vi "HostMain.vi"() -> ()   [LabVIEW 2012]
uses:
  Support VIs/operationModes.ctl
  <vilib>/MakerHub/KinectOne/Private/Type Defs/BodyData.ctl
  <vilib>/MakerHub/KinectOne/Private/Type Defs/ClippedEdges.ctl
  <vilib>/MakerHub/KinectOne/Private/Type Defs/HandLeftConfidence.ctl
  <vilib>/MakerHub/KinectOne/Private/Type Defs/HandLeftState.ctl
  <vilib>/MakerHub/KinectOne/Private/Type Defs/HandRightConfidence.ctl
  <vilib>/MakerHub/KinectOne/Private/Type Defs/HandRightState.ctl
  Microsoft.Kinect
  <vilib>/MakerHub/KinectOne/Private/Type Defs/LeanTrackingState.ctl
  Messages.ctl
  Support VIs/messageTypes.ctl
  GainsTDef.ctl
  Support VIs/speeds.ctl
  PolarCoordTdef.ctl
  Support VIs/setpointCluster.ctl
  StopTDef.ctl
  <vilib>/MakerHub/PS4-Controller/Public/Open First Controller.vi
  <vilib>/MakerHub/KinectOne/Private/Initialize Image [Color].vi
  <vilib>/MakerHub/KinectOne/Private/kinectRead [ColorFrame].vi
  <vilib>/MakerHub/KinectOne/Private/kinectRead [BodyFrame].vi
  <vilib>/MakerHub/KinectOne/KinectOne.lvlib
  <vilib>/MakerHub/PS4-Controller/LMH-PS4.lvlib
panel:
  in  "colour mode (T = dist, F = sphere)":bool
  out "Detected Colour":u32(colorbox)
  out "Tracked?":bool
  in  "Forward Speed Limit [rad/s] (10 r/s)":dbl(knob)=2.995028509599303 scale=0.0..10.0
  out "Parameter Closed":bool
  out "Kinect Closed":bool
  out "Ctrl Event Loop Off":bool
  out "Controller Off":bool
  out "Hand Ctrl Closed":bool
  out "Message Sender Closed":bool
  in  "ControllerStop":bool
  out "Controller?":bool
  out "Toggle":bool
  in  "Skynet\nButton":bool
  out "TX":bool
  in  "bodyData":T1[](array[typedef])
  in  "Modulus SP":dbl=1.7999999523162842
  in  "Reference\nColour":u32(colorbox)
  in  "Argument SP":dbl
  out "index":i32
  in  "Operation Mode":T8 items=["TeleOp", "Desperate", "ColourMatch"]
  out "Image":T9(plugin-control)
  in  "Kd-Argument":dbl
  in  "Kc-Argument":dbl=0.30000001192092896
  in  "Kd-Modulus":dbl
  in  "Kc-Modulus":dbl=0.5
  out "Mod":dbl
  out "Arg":dbl
  in  "Program Stop":bool
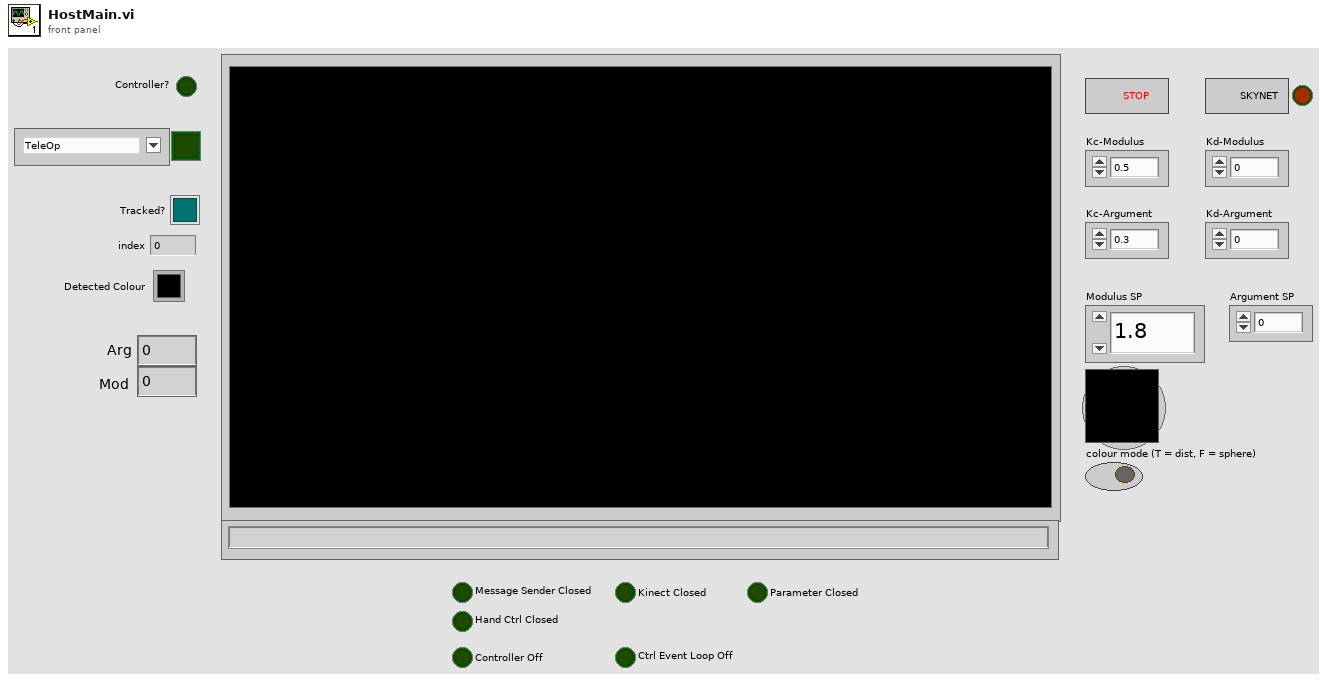
[diagram p1: front panel]
types:
  T1 = typedef "KinectOne.lvlib/BodyData.ctl" = cluster{"ClippedEdges":T2, "HandLeftConfidence":T3, "HandLeftState":T4, "HandRightConfidence":T5, "HandRightState":T6, "IsRestricted":bool, "IsTracked":bool, "JointOrientations":refnum<k24>, "Joints":refnum<k24>, "Lean":refnum<k24>, "LeanTrackingState":T7, "TrackingId":u64}
  T2 = typedef "KinectOne.lvlib/ClippedEdges.ctl" = enum16{"None", "Right", "Left", "Top", "Bottom"}
  T3 = typedef "KinectOne.lvlib/HandLeftConfidence.ctl" = enum16{"Low", "High"}
  T4 = typedef "KinectOne.lvlib/HandLeftState.ctl" = enum16{"Unknown", "NotTracked", "Open", "Closed", "Lasso"}
  T5 = typedef "KinectOne.lvlib/HandRightConfidence.ctl" = enum16{"Low", "High"}
  T6 = typedef "KinectOne.lvlib/HandRightState.ctl" = enum16{"Unknown", "NotTracked", "Open", "Closed", "Lasso"}
  T7 = typedef "KinectOne.lvlib/LeanTrackingState.ctl" = enum16{"NotTracked", "Inferred", "Tracked"}
  T8 = typedef "operationModes.ctl" = u16
  T9 = typedef "IMAQ Image.ctl" = refnum<image>
  T10 = typedef "GainsTDef.ctl" = cluster{"Kp-Modulus":dbl, "Kd-Modulus":dbl, "Kp-Argument":dbl, "Kd-Argument":dbl}
  T11 = typedef "Messages.ctl" = cluster{"message data":variant, "message type":T12}
  T12 = typedef "messageTypes.ctl" = enum16{"Speeds", "Stop", "PolarCoordinates", "Gains", "Setpoints"}
  T13 = typedef "KinectOne.lvlib/KinectSensor References.ctl" = cluster{"KinectSensor":refnum<k24>, "MultiSourceFrameReader":refnum<k24>, "BodyFrameDataInterface":refnum<k24>}
  T14 = typedef "LMH-PS4.lvlib/PS4 Controller Ref.ctl" = cluster{"Controller Ref":refnum<k1>, "PS4 Events Ref":refnum<event-registration>, "Worker Ref":refnum<vi>}
  T15 = typedef "speeds.ctl" = cluster{"left motor [rad/s]":dbl, "right motor [rad/s]":dbl}
  T16 = typedef "PolarCoordTdef.ctl" = cluster{"Argument":dbl, "Modulus":dbl, "trackedState":bool}
  T17 = typedef "KinectOne.lvlib/Joint Position.ctl" = cluster{"Camera Space":cluster{"X":dbl, "Y":dbl, "Z":dbl}, "Color Space":cluster{"X":dbl, "Y":dbl}, "Depth Space":cluster{"X":dbl, "Y":dbl}, "Tracking State":enum16{"NotTracked", "Inferred", "Tracked"}}
  T18 = typedef "setpointCluster.ctl" = cluster{"Modulus Setpoint":dbl, "Argument Setpoint":dbl}
  T19 = typedef "StopTDef.ctl" = cluster{"stop":bool}
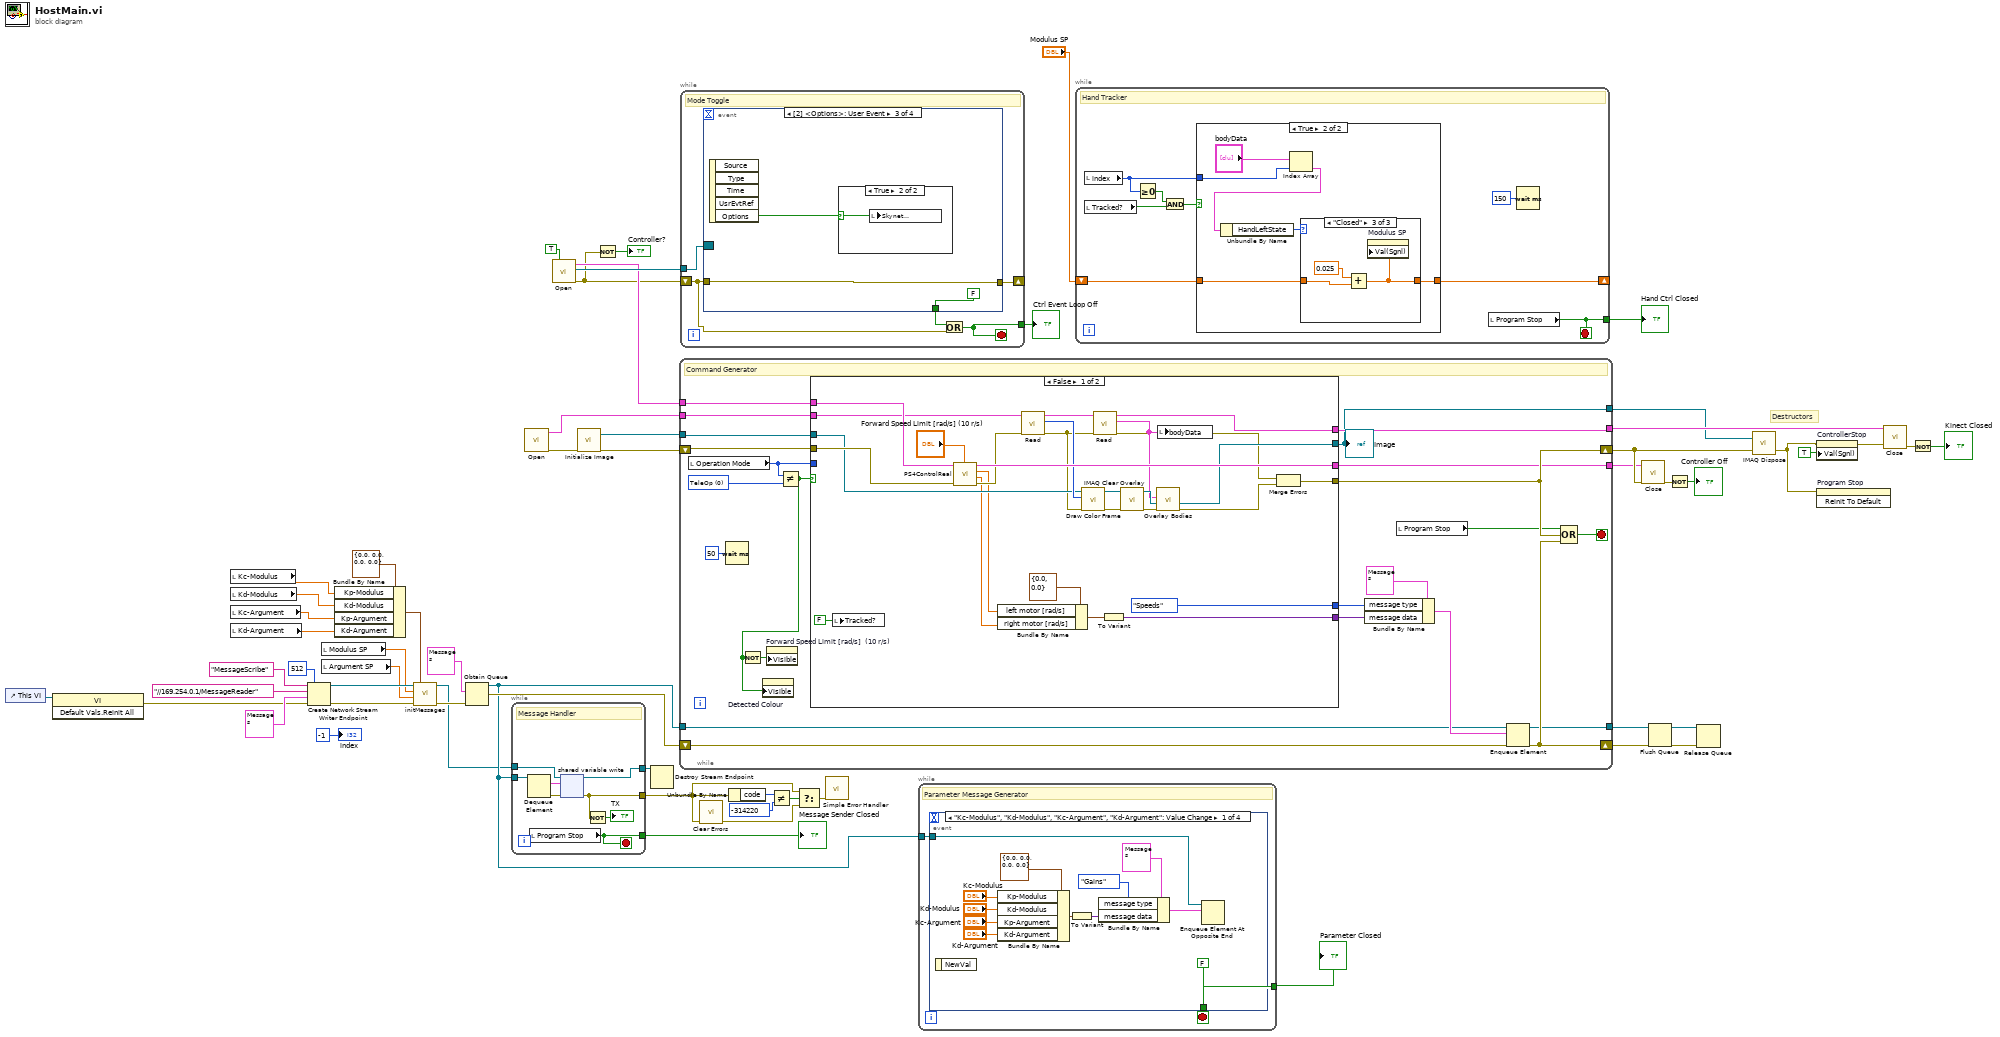
[diagram p0: block diagram]
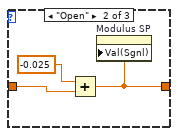
[diagram p4: hidden frame]
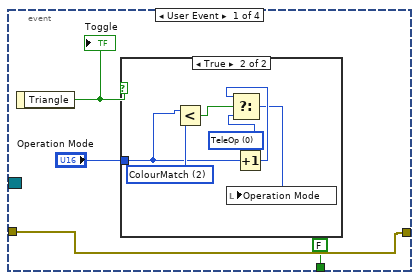
[diagram p5: hidden frame]
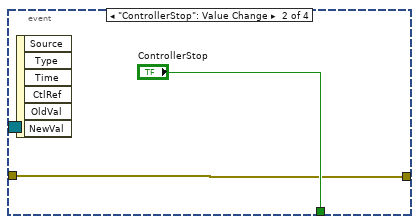
[diagram p7: hidden frame]
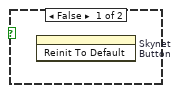
[diagram p8: hidden frame]
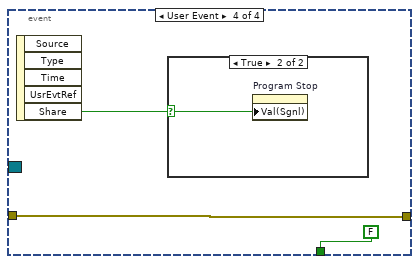
[diagram p9: hidden frame]
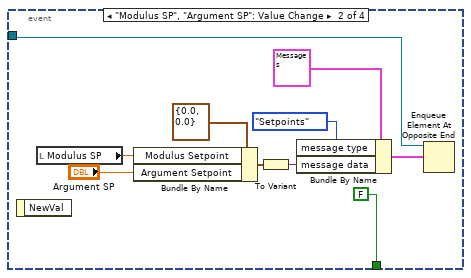
[diagram p11: hidden frame]
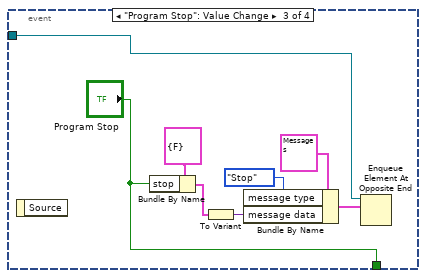
[diagram p12: hidden frame]
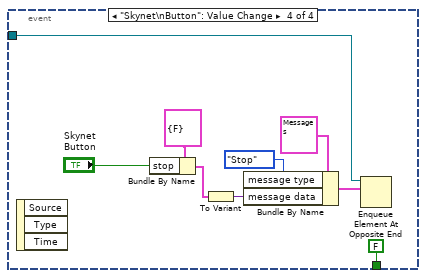
[diagram p13: hidden frame]
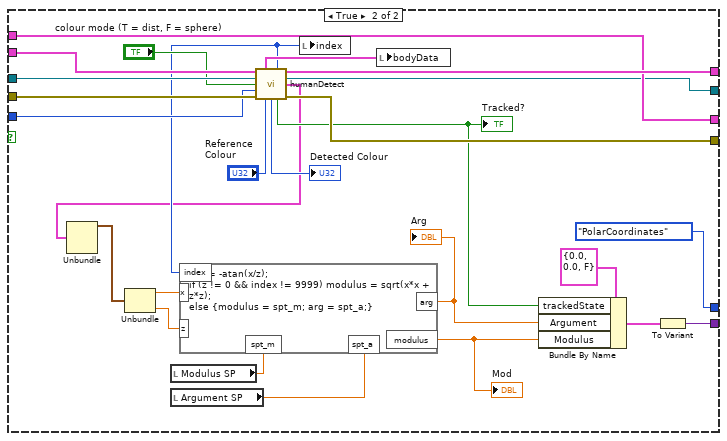
[diagram p14: hidden frame]
diagram:
  # "Destructors"
  n1 = control-ref of="This VI"() -> (w7:refnum<vi>)
  n2 = invoke class="VI" method="Default Vals.Reinit All"(reference=w7) -> (error out=w2:errorcluster)  [unwired: 2 in, 2 out]
  n3 = local read "Kc-Modulus"() -> (w30:dbl)
  n4 = local read "Kd-Modulus"() -> (w29:dbl)
  n5 = local read "Kc-Argument"() -> (w28:dbl)
  n6 = local read "Kd-Argument"() -> (w27:dbl)
  n7 = Create Network Stream Writer Endpoint(7:512 ("writer buffer size"), 8:w2, 9:T11 {"message data"=variant, "message type"=enum."Setpoints"} ("message"), 10:"//169.254.0.1/MessageReader" ("reader url"), 11:"MessageScribe" ("writer name")) -> (0:w3:errorcluster, 3:w25:refnum<k21>)  [unwired: 2 in]
  n8 = local read "Modulus SP"() -> (w24:dbl)
  n9 = local read "Argument SP"() -> (w23:dbl)
  n10 = Bundle By Name(cluster=T10 {"Kp-Modulus"=0.0, "Kd-Modulus"=0.0, "Kp-Argument"=0.0, "Kd-Argument"=0.0}, "Kp-Modulus"=w30, "Kd-Modulus"=w29, "Kp-Argument"=w28, "Kd-Argument"=w27) -> (w26:T10)
  n11 = call "initMessages.vi"("GainsCluster"=w26, "error in (no error)"=w3, "Argument Setpoint"=w23, "Modulus Setpoint"=w24, "writer name in"=w25) -> ("error out"=w22:errorcluster, "Refnum out"=w21:refnum<k21>)  [unwired: 5 in]
  n12 = Obtain Queue(element data type=T11 {"message data"=variant, "message type"=enum."Stop"} ("message"), error in (no error)=w22) -> (queue out=w48:refnum<queue>, error out=w54:errorcluster)  [unwired: 3 in, 1 out]
  n13 = while {
    tunnel: w48 -> [w66]
    tunnel: [w64] -> w33
    tunnel: [w63] -> w32
    tunnel: w21 -> [w61]
    tunnel: [w60] -> w9
    stop <- w60 stop-if-true
    # "Message Handler"
    n14 = Dequeue Element(queue=w66) -> (element=w65:T11, error out=w59:errorcluster)  [unwired: 2 in, 2 out]
    n15 = local read "Program Stop"() -> (w60:bool)
    n16 = shared-variable-write(w61, w59, w65) -> (w64:refnum<k21>, w63:errorcluster)  [unwired: 1 in, 1 out]
    n17 = Not(x=w63) -> (.not. x?=→"TX":bool)
  }
  "Message Sender Closed" <- w9
  n18 = call <vilib>:"Open.vi"() -> ("Error Out"=w58:errorcluster, "KinectSensor References out"=w51:T13)  [unwired: 10 in]
  n19 = call-poly <vilib>:"Open.vi"("Enable Events (T)"=TRUE) -> ("Error Out"=w20:errorcluster, "Event Registration Refnum"=w52:refnum<event-registration>, "PS4 Controller Ref"=w50:T14)  [unwired: 8 in]
  n20 = call-poly <vilib>:"Initialize Image.vi"("Error In"=w58) -> ("Error Out"=w57:errorcluster, "Color Image"=w56:T9)  [unwired: 9 in]
  n21 = Not(x=w20) -> (.not. x?=→"Controller?":bool)
  n22 = Destroy Stream Endpoint(11:w33) -> ()  [unwired: 1 in, 1 out]
  n23 = while {
    tunnel: w51 -> [w84]
    tunnel: w56 -> [w83]
    shift-right: [w82] -> w15
    shift-left: w57 -> [w81]
    tunnel: [w80] -> w55
    tunnel: w48 -> [w85]
    tunnel: [w72] -> w45
    tunnel: w50 -> [w79]
    tunnel: [w78] -> w14
    shift-right: [w86] -> w44
    shift-left: w54 -> [w87]
    tunnel: [w67] -> w1
    stop <- w89 stop-if-true
    w74 = T8 0 items=["TeleOp", "Desperate", "ColourMatch"] ("y")
    # "Command Generator"
    n24 = local read "Operation Mode"() -> (w75:T8)
    n25 = Wait (ms)(milliseconds to wait=u32 50) -> ()  [unwired: 1 out]
    n26 = Not Equal?(x=w75, y=w74) -> (x != y?=w70:bool)
    n27 = Not(x=w70) -> (.not. x?=w69:bool)
    n28 = property on="Detected Colour" class="ColBox"("Visible"=w70) -> ()  [unwired: 2 in, 2 out]
    n29 = property on="Forward Speed Limit [rad/s]  (10 r/s)" class="Knob (strict)"("Visible"=w69) -> ()  [unwired: 2 in, 2 out]
    n30 = case shown="False" w70 {
      tunnel: w84 -> [w113 w140]
      tunnel: w83 -> [w111 w139]
      tunnel: [w91 w138] -> w82
      tunnel: w81 -> [w115 w137]
      tunnel: [w98 w136] -> w80
      tunnel: w79 -> [w116 w129]
      tunnel: [w114 w129] -> w78
      tunnel: w75 -> [_ w133]
      tunnel: [messageTypes."Speeds" ("message type") messageTypes."PolarCoordinates" ("message type")] -> w77
      tunnel: [w105 w131] -> w76
      tunnel: [w97 w117] -> w67
      frame False {
        n31 = local write "Tracked?"(FALSE) -> ()
        n32 = call "PS4ControlReal.vi"("Forward Speed Limit [rad/s] (10.7 r/s)"="Forward Speed Limit [rad/s] (10 r/s)", "Error In"=w115, "PS4 Controller Ref In"=w116) -> ("Error Out"=w110:errorcluster, "right motor out"=w108:dbl, "left motor out"=w109:dbl, "PS4 Controller Ref Out"=w114:T14)  [unwired: 5 in]
        n33 = Bundle By Name(cluster=T15 {"left motor [rad/s]"=0.0, "right motor [rad/s]"=0.0}, "left motor [rad/s]"=w109, "right motor [rad/s]"=w108) -> (w106:T15)
        n34 = call-poly <vilib>:"Read.vi"("Error In"=w110, "KinectSensor References in"=w113) -> ("Error Out"=w95:errorcluster, "frameData"=w112:u32[], "KinectSensor References out"=w99:T13)  [unwired: 7 in]
        n35 = call <vilib>:"Draw Color Frame.vi"("Error In"=w95, "U32 Array"=w112, "Image"=w111) -> ("Error Out"=w94:errorcluster, "Image Out"=w101:T9)  [unwired: 7 in]
        n36 = call-poly <vilib>:"Read.vi"("error in (no error)"=w95, "KinectSensor References in"=w99) -> ("error out"=w92:errorcluster, "Body Data"=w96:T1[], "KinectSensor References out"=w98:T13)  [unwired: 7 in]
        n37 = To Variant(anything=w106) -> (Variant=w105:variant)
        n38 = call "IMAQ Clear Overlay"("error in (no error)"=w94, "Image"=w101) -> ("error out"=w93:errorcluster, "Image Out"=w100:T9)  [unwired: 8 in]
        n39 = call <vilib>:"Overlay Bodies.vi"("Error In"=w93, "Image"=w100, "Body Data"=w96) -> ("Error Out"=w90:errorcluster, "Image Out"=w97:T9)  [unwired: 7 in]
        n40 = local write "bodyData"(w96) -> ()
        n41 = Merge Errors(w92, w90) -> (w91:errorcluster)
      }
      frame True {
        n42 = local read "Modulus SP"() -> (w123:dbl)
        n43 = local read "Argument SP"() -> (w135:dbl)
        n44 = call "humanDetect.vi"("KinectSensor References In"=w140, "Image Container"=w139, "Tolerance Mode"="colour mode (T = dist, F = sphere)", "Operation Mode"=w133, "Error In"=w137, "Reference Colour"="Reference\nColour") -> ("Body Data Out"=w128:T1[], "Index Out"=w124:i32, "KinectSensor References Out"=w136:T13, "Image Out"=w117:T9, "Joint Position Out"=w118:T17, "Averaged Colour"=→"Detected Colour":u32, "isTracked"=w127:bool, "Error Out"=w138:errorcluster)  [unwired: 2 in]
        "Tracked?" <- w127
        n45 = Unbundle(w118) -> ("Camera Space"=w142:cluster{"X":dbl, "Y":dbl, "Z":dbl})  [unwired: 3 out]
        n46 = Unbundle(w142) -> ("X"=w120:dbl, "Z"=w119:dbl)  [unwired: 1 out]
        n47 = formula code="arg = -atan(x/z);\nif (z != 0 && index != 9999) modulus = sqrt(x*x + z*z);\nelse {modulus = spt_m; arg = spt_a;}"("x"=w120, "z"=w119, "spt_m"=w123, "spt_a"=w135, "index"=w124) -> ("arg"=w122:dbl, "modulus"=w121:dbl)
        "Arg" <- w122
        "Mod" <- w121
        n48 = local write "index"(w124) -> ()
        n49 = local write "bodyData"(w128) -> ()
        n50 = Bundle By Name(cluster=T16 {"Argument"=0.0, "Modulus"=0.0, "trackedState"=FALSE}, "trackedState"=w127, "Argument"=w122, "Modulus"=w121) -> (w132:T16)
        n51 = To Variant(anything=w132) -> (Variant=w131:variant)
      }
    }
    "Image" <- w67
    n52 = Bundle By Name(cluster=T11 {"message data"=variant, "message type"=enum."Stop"} ("message"), "message type"=w77, "message data"=w76) -> (w88:T11)
    n53 = local read "Program Stop"() -> (w68:bool)
    n54 = Enqueue Element(queue=w85, element=w88, error in (no error)=w87) -> (queue out=w72:refnum<queue>, error out=w86:errorcluster)  [unwired: 1 in, 1 out]
    n55 = Compound Arithmetic op=OR(w68, w82, w86) -> (w89:bool)
  }
  n56 = while {
    tunnel: w52 -> [w147]
    tunnel: [w143] -> w10
    shift-right: [w146] -> _
    shift-left: w20 -> [w144]
    stop <- w143 stop-if-true
    # "Mode Toggle"
    n57 = event shown="[2] <Options>: User Event" {
      selector: w147 -> [_ _ _ _]
      dyn-events: _ -> [_ _ _ _]
      timeout: _ -> [_ _ _ _]
      tunnel: w144 -> [w149 w158 w161 w165]
      tunnel: [w149 w158 w161 w165] -> w146
      tunnel: [FALSE ("ControllerStop") "ControllerStop" FALSE ("ControllerStop") FALSE ("ControllerStop")] -> w145
      event User Event {
        n58 = event-data() -> ("Triangle"=w151:bool)  [unwired: 1 in]
        "Toggle" <- w151
        n59 = case shown="True" w151 {
          tunnel: "Operation Mode" -> [_ w152]
          frame False {
          }
          frame True {
            w153 = T8 2 items=["TeleOp", "Desperate", "ColourMatch"] ("Operation Mode 2")
            w154 = T8 0 items=["TeleOp", "Desperate", "ColourMatch"] ("Operation Mode 2")
            n60 = Less?(x=w152, y=w153) -> (x < y?=w157:bool)
            n61 = Increment(x=w152) -> (x+1=w156:T8)
            n62 = Select(t=w156, s=w157, f=w154) -> (s? t:f=w155:T8)
            n63 = local write "Operation Mode"(w155) -> ()
          }
        }
      }
      event "ControllerStop": Value Change {
        n64 = event-data() -> ()  [unwired: 1 in, 6 out]
      }
      event User Event {
        n65 = event-data() -> ("Options"=w162:bool)  [unwired: 1 in, 4 out]
        n66 = case shown="True" w162 {
          selector: w162 -> [_ w163]
          frame False {
            n67 = invoke on="Skynet\nButton" class="Bool (strict)" method="Reinit To Default"() -> ()  [unwired: 3 in, 3 out]
          }
          frame True {
            n68 = local write "Skynet\nButton"(w163) -> ()
          }
        }
      }
      event User Event {
        n69 = event-data() -> ("Share"=w166:bool)  [unwired: 1 in, 4 out]
        n70 = case shown="True" w166 {
          selector: w166 -> [_ w167]
          frame False {
          }
          frame True {
            n71 = property on="Program Stop" class="Bool (strict)"("Val(Sgnl)"=w167) -> ()  [unwired: 2 in, 2 out]
          }
        }
      }
    }
    n72 = Or(x=w145, y=w144) -> (x .or. y?=w143:bool)
  }
  "Ctrl Event Loop Off" <- w10
  n73 = call <vilib>:"Clear Errors.vi"("error in (no error)"=w32) -> ("error out"=w40:errorcluster)  [unwired: 6 in]
  n74 = Unbundle By Name(w32) -> ("code"=w41:i32)
  n75 = Not Equal?(x=w41, y=-314220) -> (x != y?=w43:bool)
  n76 = Select(t=w32, s=w43, f=w40) -> (s? t:f=w34:errorcluster)
  n77 = call <vilib>:"Simple Error Handler.vi"("error in (no error)"=w34) -> ()  [unwired: 4 in, 5 out]
  n78 = while {
    tunnel: w48 -> [w169]
    tunnel: [w168] -> w8
    stop <- w168 stop-if-true
    # "Parameter Message Generator"
    n79 = event shown="[0] \"Kc-Modulus\", \"Kd-Modulus\", \"Kc-Argument\", \"Kd-Argument\": Value Change" {
      selector: _ -> [_ _ _ _]
      dyn-events: _ -> [_ _ _ _]
      timeout: _ -> [_ _ _ _]
      tunnel: w169 -> [w173 w183 w193 w202]
      tunnel: [FALSE FALSE "Program Stop" FALSE ("IT'S TIME TO")] -> w168
      event "Kc-Modulus", "Kd-Modulus", "Kc-Argument", "Kd-Argument": Value Change {
        n80 = event-data() -> ()  [unwired: 1 in, 1 out]
        n81 = Bundle By Name(cluster=T10 {"Kp-Modulus"=0.0, "Kd-Modulus"=0.0, "Kp-Argument"=0.0, "Kd-Argument"=0.0} ("GainsCluster"), "Kp-Modulus"="Kc-Modulus", "Kd-Modulus"="Kd-Modulus", "Kp-Argument"="Kc-Argument", "Kd-Argument"="Kd-Argument") -> (w177:T10)
        n82 = To Variant(anything=w177) -> (Variant=w176:variant)
        n83 = Bundle By Name(cluster=T11 {"message data"=variant, "message type"=enum."Stop"} ("message"), "message type"=messageTypes."Gains", "message data"=w176) -> (w174:T11)
        n84 = Enqueue Element At Opposite End(queue=w173, element=w174) -> ()  [unwired: 2 in, 3 out]
      }
      event "Modulus SP", "Argument SP": Value Change {
        n85 = event-data() -> ()  [unwired: 1 in, 1 out]
        n86 = local read "Modulus SP"() -> (w189:dbl)
        n87 = Bundle By Name(cluster=T18 {"Modulus Setpoint"=0.0, "Argument Setpoint"=0.0} ("Setpoint Cluster"), "Modulus Setpoint"=w189, "Argument Setpoint"="Argument SP") -> (w188:T18)
        n88 = To Variant(anything=w188) -> (Variant=w186:variant)
        n89 = Bundle By Name(cluster=T11 {"message data"=variant, "message type"=enum."Stop"} ("message"), "message type"=messageTypes."Setpoints", "message data"=w186) -> (w187:T11)
        n90 = Enqueue Element At Opposite End(queue=w183, element=w187) -> ()  [unwired: 2 in, 3 out]
      }
      event "Program Stop": Value Change {
        n91 = event-data() -> ()  [unwired: 1 in, 1 out]
        n92 = Bundle By Name(cluster=T19 {"stop"=FALSE} ("Cluster"), "stop"="Program Stop") -> (w199:T19)
        n93 = To Variant(anything=w199) -> (Variant=w195:variant)
        n94 = Bundle By Name(cluster=T11 {"message data"=variant, "message type"=enum."Stop"} ("message"), "message type"=messageTypes."Stop", "message data"=w195) -> (w196:T11)
        n95 = Enqueue Element At Opposite End(queue=w193, element=w196) -> ()  [unwired: 2 in, 3 out]
      }
      event "Skynet\nButton": Value Change {
        n96 = event-data() -> ()  [unwired: 1 in, 3 out]
        n97 = Bundle By Name(cluster=T19 {"stop"=FALSE} ("Cluster"), "stop"="Skynet\nButton") -> (w208:T19)
        n98 = To Variant(anything=w208) -> (Variant=w204:variant)
        n99 = Bundle By Name(cluster=T11 {"message data"=variant, "message type"=enum."Stop"} ("message"), "message type"=messageTypes."Stop", "message data"=w204) -> (w205:T11)
        n100 = Enqueue Element At Opposite End(queue=w202, element=w205) -> ()  [unwired: 2 in, 3 out]
      }
    }
  }
  "Parameter Closed" <- w8
  n101 = while {
    shift-right: [w210] -> _
    shift-left: "Modulus SP" -> [w212]
    tunnel: [w209] -> w5
    stop <- w209 stop-if-true
    # "Hand Tracker"
    n102 = local read "index"() -> (w213:i32)
    n103 = local read "Tracked?"() -> (w214:bool)
    n104 = Greater Or Equal To 0?(x=w213) -> (x >= 0?=w215:bool)
    n105 = And(x=w215, y=w214) -> (x .and. y?=w216:bool)
    n106 = case shown="True" w216 {
      tunnel: w213 -> [_ w223]
      tunnel: w212 -> [w217 w220]
      tunnel: [w217 w218] -> w210
      frame False {
      }
      frame True {
        n107 = Index Array(array="bodyData", index=w223) -> (element=w222:T1)
        n108 = Unbundle By Name(w222) -> ("HandLeftState"=w221:T4)
        n109 = case shown="\"Closed\"" w221 {
          tunnel: w220 -> [w224 w226 w229]
          tunnel: [w224 w225 w228] -> w218
          frame "Unknown", Default {
          }
          frame "Open" {
            n110 = Add(x=-0.025, y=w226) -> (x+y=w225:dbl)
            n111 = property on="Modulus SP" class="DigNum (strict)"("Val(Sgnl)"=w225) -> ()  [unwired: 2 in, 2 out]
          }
          frame "Closed" {
            n112 = Add(x=0.025, y=w229) -> (x+y=w228:dbl)
            n113 = property on="Modulus SP" class="DigNum (strict)"("Val(Sgnl)"=w228) -> ()  [unwired: 2 in, 2 out]
          }
        }
      }
    }
    n114 = local read "Program Stop"() -> (w209:bool)
    n115 = Wait (ms)(milliseconds to wait=u32 150) -> ()  [unwired: 1 out]
  }
  "Hand Ctrl Closed" <- w5
  n116 = call <vilib>:"Close.vi"("Error In"=w15, "PS4 Controller Ref"=w14) -> ("Error Out"=w4:errorcluster)  [unwired: 9 in]
  n117 = Flush Queue(queue=w45, error in (no error)=w44) -> (queue out=w47:refnum<queue>, error out=w46:errorcluster)  [unwired: 1 out]
  n118 = Not(x=w4) -> (.not. x?=→"Controller Off":bool)
  n119 = Release Queue(queue=w47, error in (no error)=w46) -> ()  [unwired: 1 in, 3 out]
  n120 = call "IMAQ Dispose"("Image"=w1, "error in (no error)"=w15) -> ("error out"=w6:errorcluster)  [unwired: 4 in]
  n121 = property on="ControllerStop" class="Bool (strict)"(error in=w6, "Val(Sgnl)"=TRUE ("Value (Signaling)")) -> (error out=w17:errorcluster)  [unwired: 1 in, 1 out]
  n122 = invoke on="Program Stop" class="Bool (strict)" method="Reinit To Default"(error in=w6) -> ()  [unwired: 2 in, 3 out]
  n123 = call <vilib>:"Close.vi"("Error In"=w17, "KinectSensor References"=w55) -> ("Error Out"=w12:errorcluster)  [unwired: 9 in]
  n124 = Not(x=w12) -> (.not. x?=→"Kinect Closed":bool)
  "index" <- -1 ("index")
